vi "Set Text Color Dialog.vi"() -> (2 "Text Color Out":u32(colorbox), 3 "Cancelled?":bool caption="取消？")   [LabVIEW 2013, in "IP Adresss Control.xctl"]
doc: "该模板用于创建能够进行事件处理的对话框。"
uses:
  IP Adresss Control.xctl
panel:
  in  "Text Color":u32(colorbox)
  in  "Cancel":bool caption="取消"
  in  "OK":bool caption="确定"
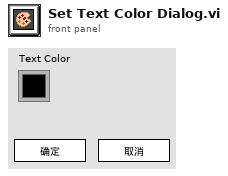
[diagram p1: front panel]
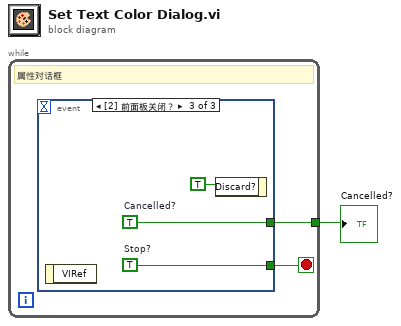
[diagram p0: block diagram]
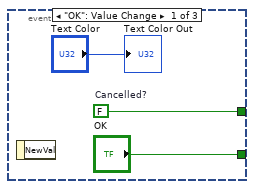
[diagram p2: hidden frame]
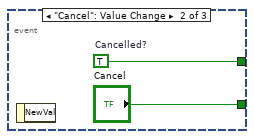
[diagram p3: hidden frame]
diagram:
  n1 = while {
    tunnel: [w2] -> w1
    stop <- w3 stop-if-true
    # "属性对话框"
    n2 = event shown="[2] 前面板关闭？" {
      selector: _ -> [_ _ _]
      dyn-events: _ -> [_ _ _]
      timeout: _ -> [_ _ _]
      tunnel: ["OK" "Cancel" w10] -> w3
      tunnel: [w6 w8 w9] -> w2
      event "OK": Value Change {
        w6 = FALSE  # Cancelled?
        n3 = event-data() -> ()  [unwired: 1 in, 1 out]
        "Text Color Out" <- "Text Color"
      }
      event "Cancel": Value Change {
        w8 = TRUE  # Cancelled?
        n4 = event-data() -> ()  [unwired: 1 in, 1 out]
      }
      event Panel Close? {
        w9 = TRUE  # Cancelled?
        w10 = TRUE  # Stop?
        n5 = event-data() -> ()  [unwired: 1 in, 1 out]
        n6 = event-data("Discard?"=TRUE) -> ()  [unwired: 1 in, 1 out]
      }
    }
  }
  "Cancelled?" <- w1
